vi "Ler_temperatura.vi"(4 "order":i32=2, 6 "intervals":i32=20, 8 "low cutoff freq: fl":dbl=0.12500000000000006 format="%0.4f", 9 "high cutoff freq: fh":dbl=0.45000000000000007 format="%0.2f", 10 "filter type":T3, 11 "Statistic":T1(ring)) -> (0 "String":string, 1 "mean value pressao":dbl, 2 "Data Set 2 Output":dbl format="%.4g", 3 "Data Set 1 Output":dbl format="%.4g")   [LabVIEW 2011]
uses:
  <vilib>/Analysis/3filter.llb/Filter Passband Type.ctl
  <vilib>/DAQmx/read.llb/DAQmx Read (Analog 1D DBL 1Chan NSamp).vi
  <vilib>/DAQmx/create/channels.llb/DAQmx Create Channel (AI-Voltage-Basic).vi
  <vilib>/DAQmx/configure/timing.llb/DAQmx Timing (Sample Clock).vi
  <vilib>/DAQmx/miscellaneous.llb/DAQmx Fill In Error Info.vi
  <vilib>/Analysis/3filter.llb/Butterworth Filter (DBL).vi
  <vilib>/Analysis/baseanly.llb/Unimode.vi
  <vilib>/Analysis/5stat.llb/RMS (DBL).vi
  Program Files/National Instruments/LabVIEW 2011/resource/objmgr/daqmx.rc
  <vilib>/gmath/NI_Gmath.lvlib
  <vilib>/Analysis/NI_AALBase.lvlib
  <vilib>/Analysis/NI_AALPro.lvlib
panel:
  out "?":T2(graph)
  out "Data Set 1":dbl[](graph)
  out "?":T2(graph)
  out "Data Set 2":dbl[](graph)
  out "error":dbl
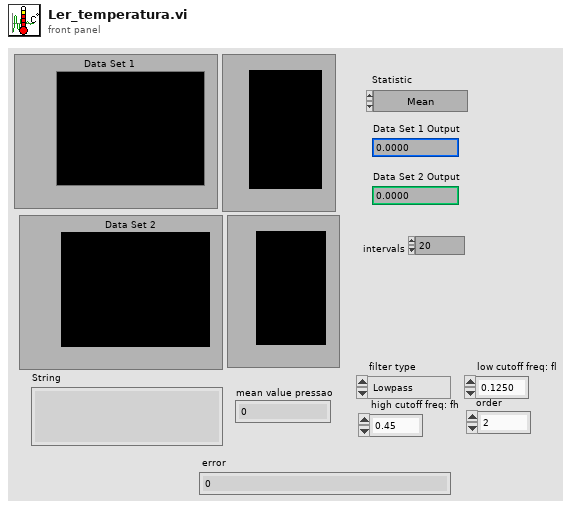
[diagram p1: front panel]
types:
  T1 = enum16{"Mean", "Standard Deviation", "Variance", "Skewness", "Kurtosis", "Median", "Mode", "RMS"}
  T2 = cluster{"Histogram: h(x)":i32[], "X Values":dbl[]}
  T3 = typedef "NI_AALBase.lvlib/Filter Passband Type.ctl" = enum32{"Lowpass", "Highpass", "Bandpass", "Bandstop"}
  T4 = enum16{"arithmetic", "geometric", "harmonic", "trimmed", "median"}
  T5 = cluster{"intervals":i32, "Statistic":enum16{"Mean", "Standard Deviation", "Variance", "Skewness", "Kurtosis", "Median", "Mode", "RMS"}}
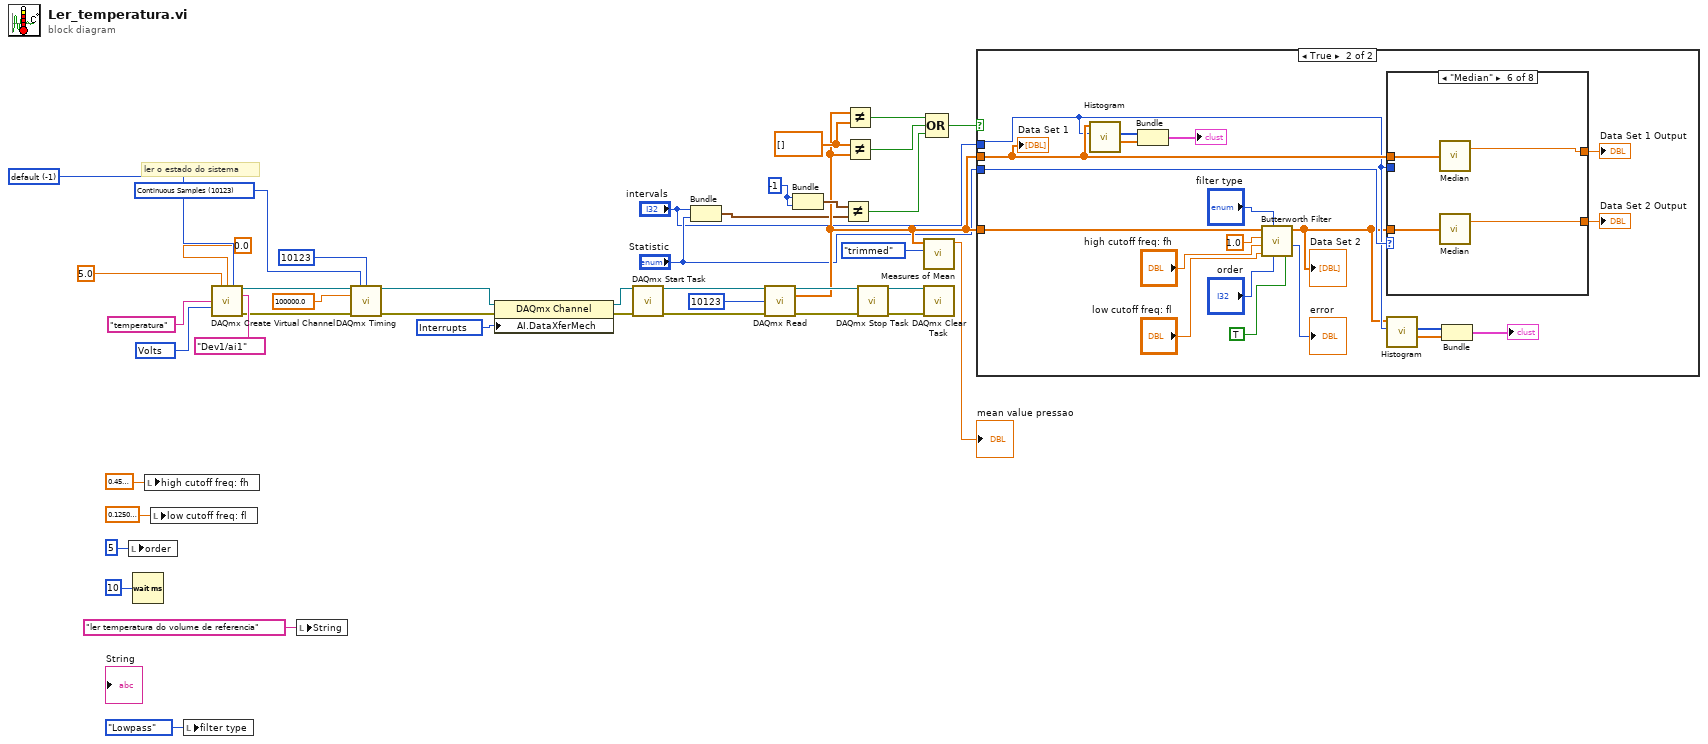
[diagram p0: block diagram]
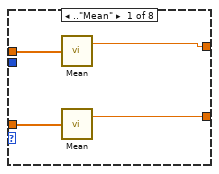
[diagram p3: hidden frame]
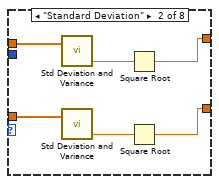
[diagram p4: hidden frame]
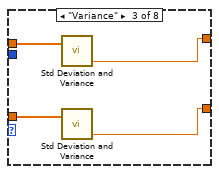
[diagram p5: hidden frame]
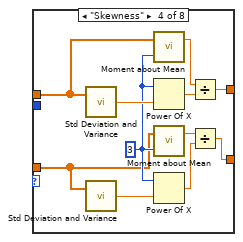
[diagram p6: hidden frame]
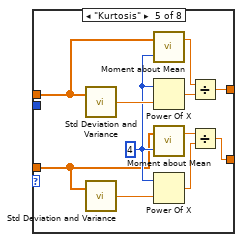
[diagram p7: hidden frame]
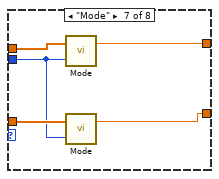
[diagram p8: hidden frame]
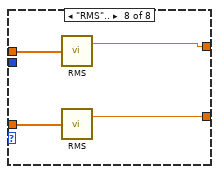
[diagram p9: hidden frame]
diagram:
  w34 = -1 items=["default"=-1, "RSE"=10083, "NRSE"=10078, "Differential"=10106, "Pseudodifferential"=12529] ("input terminal configuration")
  w11 = dbl[] []
  w9 = -1
  w27 = 10204 items=["DMA"=10054, "Interrupts"=10204, "Programmed I/O"=10264, "USB Bulk"=12590] ("AI.DataXferMech")
  w30 = 10123 items=["Finite Samples"=10178, "Continuous Samples"=10123, "Hardware Timed Single Point"=12522] ("sample mode")
  w35 = 10348 items=["Volts"=10348, "From Custom Scale"=10065] ("units")
  # "ler o estado do sistema"
  n1 = local write "order"(5 ("order")) -> ()
  n2 = Wait (ms)(milliseconds to wait=u32 10) -> ()  [unwired: 1 out]
  n3 = local write "high cutoff freq: fh"(0.45000000000000007 ("high cutoff freq: fh")) -> ()
  n4 = local write "low cutoff freq: fl"(0.12500000000000006 ("low cutoff freq: fl")) -> ()
  n5 = local write "filter type"(Filter_Passband_Type."Lowpass" ("filter type")) -> ()
  n6 = call-poly <vilib>:"DAQmx Create Virtual Channel.vi"("maximum value"=5.0, "minimum value"=0.0, "input terminal configuration"=w34, "physical channels"=tag "Dev1/ai1" ("P S1"), "name to assign"="temperatura", "units"=w35) -> ("task out"=w24:refnum<k21>, "error out"=w23:errorcluster)  [unwired: 8 in]
  n7 = local write "String"("ler temperatura do volume de referencia" ("String")) -> ()
  n8 = call-poly <vilib>:"DAQmx Timing.vi"("task/channels in"=w24, "sample mode"=w30, "samples per channel"=10123, "rate"=100000.0, "error in"=w23) -> ("task out"=w29:refnum<k21>, "error out"=w28:errorcluster)  [unwired: 9 in]
  n9 = property class="DAQmx Channel"(reference=w29, error in=w28, "AI.DataXferMech"=w27) -> (reference out=w26:refnum<k21>, error out=w25:errorcluster)
  n10 = call <vilib>:"DAQmx Start Task.vi"("task/channels in"=w26, "error in"=w25) -> ("task out"=w32:refnum<k21>, "error out"=w31:errorcluster)  [unwired: 12 in]
  n11 = Bundle("intervals"="intervals", "Statistic"="Statistic") -> (w3:T5)  [unwired: 1 in]
  n12 = call-poly <vilib>:"DAQmx Read.vi"("task/channels in"=w32, "number of samples per channel"=10123, "error in"=w31) -> ("task out"=w16:refnum<k21>, "data"=w8:dbl[], "error out"=w14:errorcluster)  [unwired: 10 in]
  n13 = Bundle(w9, w9) -> (w10:cluster{i32, i32})  [unwired: 1 in]
  n14 = Not Equal?(x=w10, y=w3) -> (x != y?=w2:bool)
  n15 = Not Equal?(x=w8, y=w11) -> (x != y?=w6:bool)
  n16 = Not Equal?(x=w11, y=w8) -> (x != y?=w5:bool)
  n17 = call <vilib>:"DAQmx Stop Task.vi"("task/channels in"=w16, "error in"=w14) -> ("task out"=w15:refnum<k21>, "error out"=w13:errorcluster)  [unwired: 12 in]
  n18 = call <vilib>:"Measures of Mean.vi"("type"=T4."trimmed", "x array"=w8) -> ("mean value"=→"mean value pressao":dbl)  [unwired: 8 in, 1 out]
  n19 = call <vilib>:"DAQmx Clear Task.vi"("task in"=w15, "error in"=w13) -> ()  [unwired: 13 in, 1 out]
  n20 = Compound Arithmetic op=OR(w6, w5, w2) -> (w7:bool)
  n21 = case shown="True" w7 {
    tunnel: w8 -> [_ w49]
    tunnel: w8 -> [_ w58]
    tunnel: "Statistic" -> [_ w60]
    tunnel: "intervals" -> [_ w56]
    frame False {
    }
    frame True {
      n22 = call <vilib>:"Histogram.vi"("intervals"=w56, "X"=w58) -> ("X Values"=w54:dbl[], "Histogram: h(x)"=w55:i32[])  [unwired: 6 in, 2 out]
      n23 = Bundle("Histogram: h(x)"=w55, "X Values"=w54) -> (→"?":T2)  [unwired: 1 in]
      n24 = call-poly <vilib>:"Butterworth Filter.vi"("init/cont (init:F)"=TRUE, "order"="order", "filter type"="filter type", "low cutoff freq: fl"="low cutoff freq: fl", "high cutoff freq: fh"="high cutoff freq: fh", "sampling freq: fs"=1.0, "X"=w49) -> ("error"=→"error":i32, "Filtered X"=w48:dbl[])  [unwired: 1 in]
      "Data Set 2" <- w48
      n25 = case shown="\"Median\"" w60 {
        tunnel: w48 -> [w66 w71 w75 w82 w93 w102 w107 w111]
        tunnel: [w64 w68 w74 w79 w90 w100 w105 w110] -> w61
        tunnel: [w65 w72 w76 w83 w94 w101 w106 w109] -> w62
        tunnel: w58 -> [w63 w67 w73 w86 w97 w99 w104 w108]
        tunnel: w56 -> [_ _ _ _ _ _ w103 _]
        frame .."Mean" {
          n26 = call <vilib>:"Mean.vi"("X"=w63) -> ("mean"=w65:dbl)  [unwired: 1 out]
          n27 = call <vilib>:"Mean.vi"("X"=w66) -> ("mean"=w64:dbl)  [unwired: 1 out]
        }
        frame "Standard Deviation" {
          n28 = call <vilib>:"Std Deviation and Variance.vi"("X"=w67) -> ("variance"=w70:dbl)  [unwired: 1 in, 2 out]
          n29 = call <vilib>:"Std Deviation and Variance.vi"("X"=w71) -> ("variance"=w69:dbl)  [unwired: 1 in, 2 out]
          n30 = Square Root(x=w70) -> (sqrt(x)=w72:dbl)
          n31 = Square Root(x=w69) -> (sqrt(x)=w68:dbl)
        }
        frame "Variance" {
          n32 = call <vilib>:"Std Deviation and Variance.vi"("X"=w73) -> ("variance"=w76:dbl)  [unwired: 1 in, 2 out]
          n33 = call <vilib>:"Std Deviation and Variance.vi"("X"=w75) -> ("variance"=w74:dbl)  [unwired: 1 in, 2 out]
        }
        frame "Skewness" {
          w84 = 3
          n34 = call <vilib>:"Std Deviation and Variance.vi"("X"=w86) -> ("standard deviation"=w87:dbl)  [unwired: 1 in, 2 out]
          n35 = call <vilib>:"Std Deviation and Variance.vi"("X"=w82) -> ("standard deviation"=w85:dbl)  [unwired: 1 in, 2 out]
          n36 = call <vilib>:"Moment about Mean.vi"("order"=w84, "X"=w86) -> ("moment"=w77:dbl)  [unwired: 1 out]
          n37 = Power Of X(1:w87, 2:w84) -> (0:w78:dbl)
          n38 = call <vilib>:"Moment about Mean.vi"("order"=w84, "X"=w82) -> ("moment"=w80:dbl)  [unwired: 1 out]
          n39 = Power Of X(1:w85, 2:w84) -> (0:w81:dbl)
          n40 = Divide(x=w77, y=w78) -> (x/y=w83:dbl)
          n41 = Divide(x=w80, y=w81) -> (x/y=w79:dbl)
        }
        frame "Kurtosis" {
          w95 = 4
          n42 = call <vilib>:"Std Deviation and Variance.vi"("X"=w97) -> ("standard deviation"=w98:dbl)  [unwired: 1 in, 2 out]
          n43 = call <vilib>:"Std Deviation and Variance.vi"("X"=w93) -> ("standard deviation"=w96:dbl)  [unwired: 1 in, 2 out]
          n44 = call <vilib>:"Moment about Mean.vi"("order"=w95, "X"=w97) -> ("moment"=w89:dbl)  [unwired: 1 out]
          n45 = Power Of X(1:w98, 2:w95) -> (0:w88:dbl)
          n46 = call <vilib>:"Moment about Mean.vi"("order"=w95, "X"=w93) -> ("moment"=w91:dbl)  [unwired: 1 out]
          n47 = Power Of X(1:w96, 2:w95) -> (0:w92:dbl)
          n48 = Divide(x=w89, y=w88) -> (x/y=w94:dbl)
          n49 = Divide(x=w91, y=w92) -> (x/y=w90:dbl)
        }
        frame "Median" {
          n50 = call <vilib>:"Median.vi"("X"=w99) -> ("median"=w101:dbl)  [unwired: 1 out]
          n51 = call <vilib>:"Median.vi"("X"=w102) -> ("median"=w100:dbl)  [unwired: 1 out]
        }
        frame "Mode" {
          n52 = call-poly <vilib>:"Mode.vi"("intervals"=w103, "X"=w104) -> ("mode"=w106:dbl)  [unwired: 1 out]
          n53 = call-poly <vilib>:"Mode.vi"("intervals"=w103, "X"=w107) -> ("mode"=w105:dbl)  [unwired: 1 out]
        }
        frame "RMS".. {
          n54 = call-poly <vilib>:"RMS.vi"("X"=w108) -> ("rms value"=w109:dbl)  [unwired: 1 out]
          n55 = call-poly <vilib>:"RMS.vi"("X"=w111) -> ("rms value"=w110:dbl)  [unwired: 1 out]
        }
      }
      "Data Set 1 Output" <- w62
      "Data Set 2 Output" <- w61
      n56 = call <vilib>:"Histogram.vi"("intervals"=w56, "X"=w48) -> ("X Values"=w52:dbl[], "Histogram: h(x)"=w53:i32[])  [unwired: 6 in, 2 out]
      n57 = Bundle("Histogram: h(x)"=w53, "X Values"=w52) -> (→"?":T2)  [unwired: 1 in]
      "Data Set 1" <- w58
    }
  }
